vi "ConvertToArrayCMP.vi"(8 "error in (no error)":errorcluster, 11 "Cluster":T1) -> (0 "error out":errorcluster, 3 "Array":dbl[](array[numeric]))   [LabVIEW 2014]
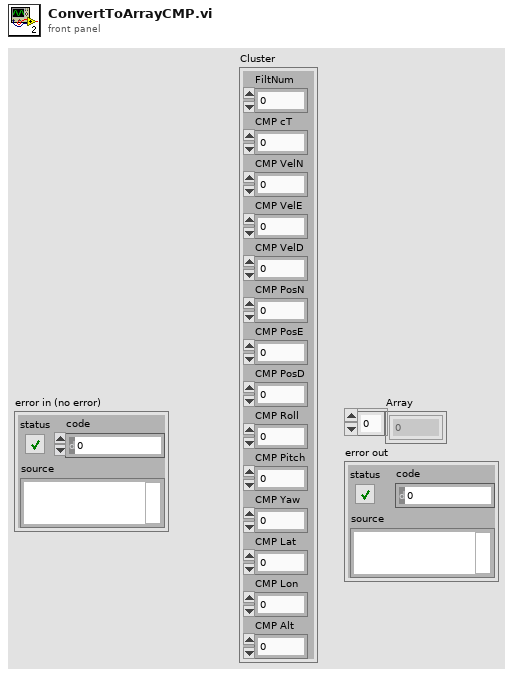
[diagram p1: front panel]
types:
  T1 = cluster{"FiltNum":i32, "CMP cT":dbl, "CMP VelN":sgl, "CMP VelE":sgl, "CMP VelD":sgl, "CMP PosN":sgl, "CMP PosE":sgl, "CMP PosD":sgl, "CMP Roll":sgl, "CMP Pitch":sgl, "CMP Yaw":sgl, "CMP Lat":dbl, "CMP Lon":dbl, "CMP Alt":sgl}
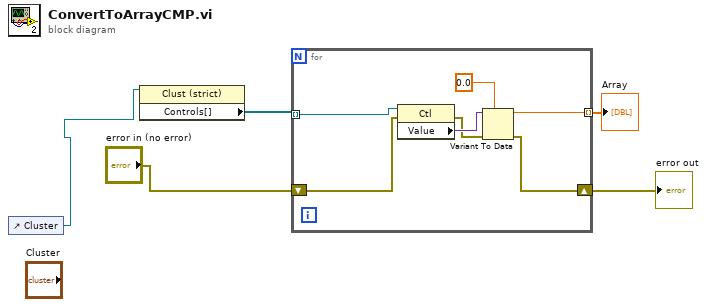
[diagram p0: block diagram]
diagram:
  n1 = control-ref of="Cluster"() -> (w1:refnum<vi>)
  n2 = property class="Clust (strict)"(reference=w1) -> ("Controls[]"=w2:refnum<vi>[])  [unwired: 1 in, 2 out]
  n3 = for {
    tunnel: w2 -> [w12] mode=indexing
    tunnel: [w9] -> w5 mode=indexing
    shift-right: [w6] -> w3
    shift-left: "error in (no error)" -> [w7]
    n4 = property class="Ctl"(reference=w12, error in=w7) -> (error out=w8:errorcluster, "Value"=w11:variant)  [unwired: 1 out]
    n5 = Variant To Data(error in=w8, type=0.0, Variant=w11) -> (data=w9:dbl, error out=w6:errorcluster)
  }
  "Array" <- w5
  "error out" <- w3
